vi "Actor Core.vi"(8 "error in":errorcluster, 11 "State in":refnum<class "State Actor.lvclass">) -> (0 "error out":errorcluster, 3 "Actor out":refnum<class "Actor.lvclass">)   [LabVIEW 2020, in "State Actor.lvclass"]
doc: "(<B>Filename</B>: Actor Framework.lvlib:Actor.lvclass:Actor Core.vi)\n\nThis override invokes Entry.vi on the initial state, prior to calling the parent Actor Core. Adding this behavior to Actor Core (instead of an override of Pre Launch Init.vi) allows the initial state to launch a nested actor as part of its entry behavior.\n\nReceives messages to the actor, reacts to them, and initiates any error handling that may shut the actor down.\n\nDescendant classes may override this VI to append parallel tasks for the actor to complete while it handles messages. Overrides use the Call Parent Method node."
uses:
  State Actor.lvclass
  C:/Program Files (x86)/National Instruments/LabVIEW 2020/vi.lib/ActorFramework/Actor/Actor.lvclass
  <vilib>/ActorFramework/Actor/Actor.lvclass
  State Actor.lvclass/State Actor.ctl
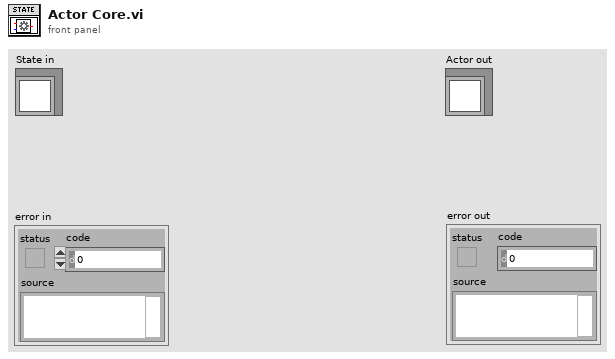
[diagram p1: front panel]
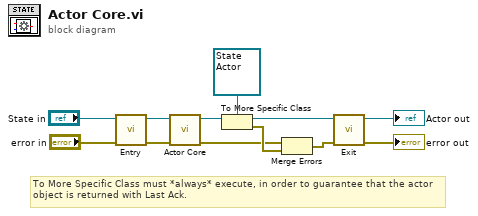
[diagram p0: block diagram]
diagram:
  # "To More Specific Class must *always* execute, in order to guarantee that the actor object is returned with Last Ack."
  n1 = call-dynamic "Entry.vi"("error in (no error)"="error in", "New State"="State in") -> ("error out"=w9:errorcluster, "State out"=w10:refnum<class "State Actor.lvclass">)  [unwired: 8 in]
  n2 = call-parent "Actor Core.vi"("error in"=w9, "Actor in"=w10) -> ("error out"=w1:errorcluster, "Actor out"=w7:refnum<class "Actor.lvclass">)  [unwired: 8 in]
  n3 = To More Specific Class(target class=refnum<class "State Actor.lvclass"> refnum ("State in"), reference=w7) -> (specific class reference=w6:refnum<class "State Actor.lvclass">, error out=w8:errorcluster)  [unwired: 1 in]
  n4 = Merge Errors(w1, w8) -> (w2:errorcluster)
  n5 = call-dynamic "Exit.vi"("error in (no error)"=w2, "Old State"=w6) -> ("error out"=→"error out":errorcluster, "New State"=→"Actor out":refnum<class "State Actor.lvclass">)  [unwired: 8 in]
